vi "Start Server.vi"(8 "error in":errorcluster, 11 "gRPC Server in":refnum<class "Servicer.lvclass">) -> (0 "error out":errorcluster, 2 "Listening Port":i32, 3 "gRPC Server out":refnum<class "Servicer.lvclass">)   [LabVIEW 2019, in "gRPC-servicer.lvlib" / "Servicer.lvclass"]
uses:
  Servicer.lvclass
  Servicer.lvclass/Servicer.ctl
  gRPC lv Support/grpc-lvsupport/grpc-lvsupport.lvlib
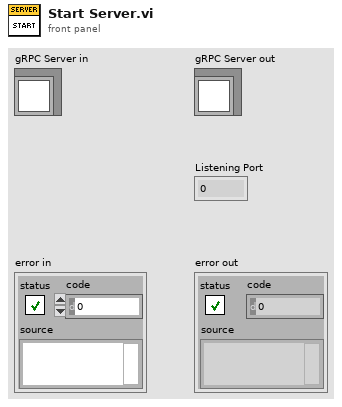
[diagram p1: front panel]
types:
  T1 = typedef "grpc-lvsupport.lvlib/grpcId.ctl" = u64
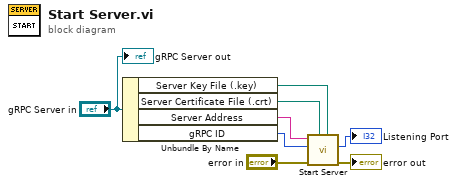
[diagram p0: block diagram]
diagram:
  n1 = Unbundle By Name("gRPC Server in") -> ("Server Key File (.key)"=w3:path, "Server Certificate File (.crt)"=w2:path, "Server Address"=w4:string, "gRPC ID"=w1:T1)
  n2 = call "Start Server.vi"("Server Key File (.key)"=w3, "Server Certificate File (.crt)"=w2, "error in"="error in", "gRPCid server in"=w1, "Server Address"=w4) -> ("error out"=→"error out":errorcluster, "Listening Port"=→"Listening Port":i32)  [unwired: 4 in, 1 out]
  "gRPC Server out" <- "gRPC Server in"
